vi "Unflatten Value.vi"(8 "Error In":errorcluster, 10 "Value":string, 11 "Path Array In":refnum<class "1D Path.lvclass">) -> (0 "Error Out":errorcluster, 3 "Path Array Out":refnum<class "1D Path.lvclass">)   [LabVIEW 2017, in "Tree API.lvlib" / "1D Path.lvclass"]
uses:
  1D Path.lvclass
  Tree Manager/Tree.lvclass
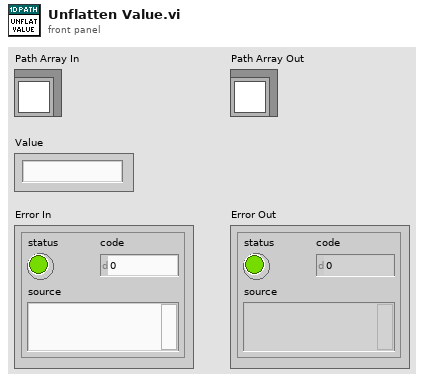
[diagram p1: front panel]
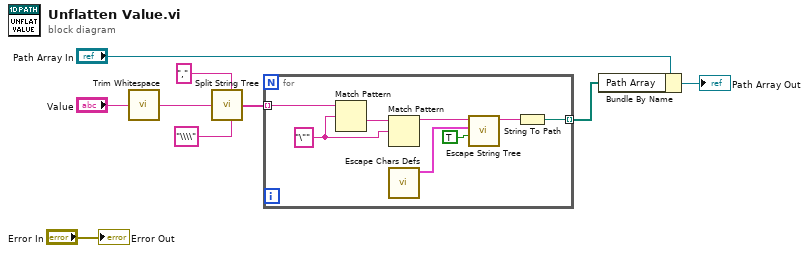
[diagram p0: block diagram]
diagram:
  n1 = call <vilib>:"Trim Whitespace.vi"("string"="Value") -> ("trimmed string"=w1:string)  [unwired: 1 in]
  n2 = call "Split String Tree.vi"("Ignore Pattern"="\\\\", "Split Pattern"=",", "Input String"=w1) -> ("Split String"=w7:string[])  [unwired: 4 in]
  n3 = for {
    tunnel: w7 -> [w16] mode=indexing
    tunnel: [w17] -> w5 mode=indexing
    w14 = "\"" ("regular expression")
    n4 = Match Pattern(string=w16, regular expression=w14) -> (after substring=w15:string)  [unwired: 1 in, 3 out]
    n5 = Match Pattern(string=w15, regular expression=w14) -> (before substring=w12:string)  [unwired: 1 in, 3 out]
    n6 = call "Escape Chars Defs.vi"() -> ("Escapes"=w13:cluster{"String":string, "Escape":string}[])  [unwired: 11 in]
    n7 = call "Escape String Tree.vi"("Reverse? (False)"=TRUE, "Escapes"=w13, "String In"=w12) -> ("String Out"=w11:string)  [unwired: 8 in]
    n8 = String To Path(string=w11) -> (path=w17:path)
  }
  n9 = Bundle By Name(cluster="Path Array In", "Path Array"=w5) -> (→"Path Array Out":refnum<class "1D Path.lvclass">)
  "Error Out" <- "Error In"
